vi "motor encoder.vi"(8 "Error In":errorcluster, 9 "motor select":T2, 10 "Reset":bool, 11 "FPGA VI Reference In":T1) -> (0 "error out":errorcluster, 1 "encoder":i32, 3 "FPGA VI Reference Out":T1)   [LabVIEW 2019, in "my FPGA lib.lvlib" / "motor.lvlib"]
uses:
  motor.lvlib
  motor enum.ctl
  FPGA/FPPGA.ctl
  <vilib>/Utility/error.llb/Error Cluster From Error Code.vi
  <vilib>/rvi/errors/niLvFpgaAdjustHostInterfaceError.vi
  <vilib>/rvi/interface/nirviReadWriteControl/nirviReadWriteControl.xnode
  NiFpgaLv.dll
  <vilib>/rvi/interface/Simulation/niFpgaSimulationCallBeginRW.vi
  my FPGA lib.lvlib
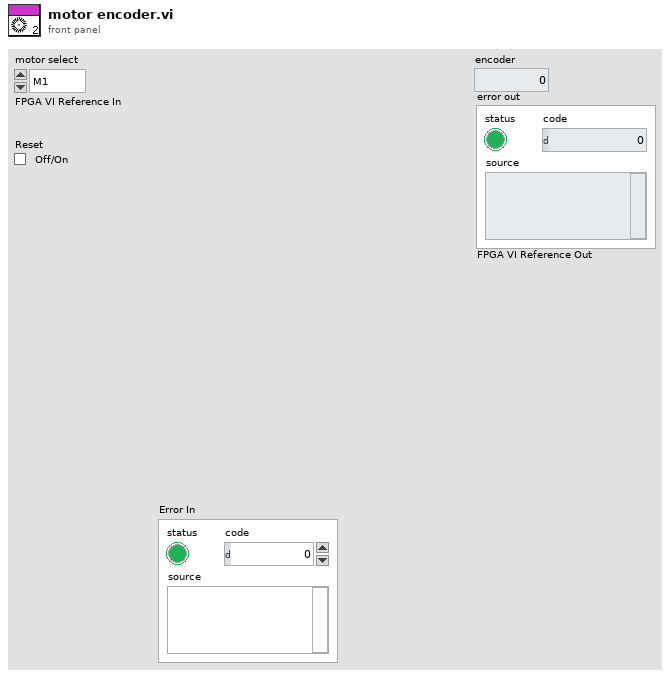
[diagram p1: front panel]
types:
  T1 = typedef "my FPGA lib.lvlib/FPPGA.ctl" = refnum<k20>
  T2 = typedef "my FPGA lib.lvlib/motor.lvlib/motor enum.ctl" = enum16{"M1", "M2", "M3", "M4"}
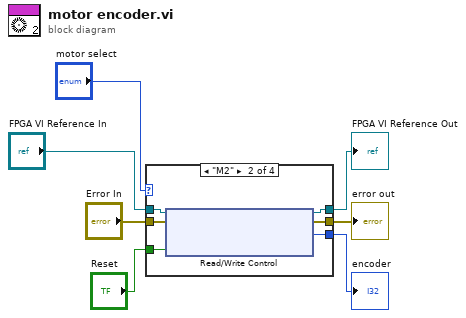
[diagram p0: block diagram]
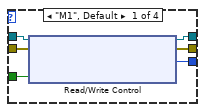
[diagram p2: hidden frame]
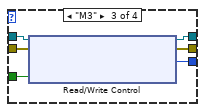
[diagram p3: hidden frame]
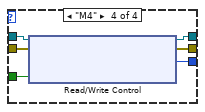
[diagram p4: hidden frame]
diagram:
  n1 = case shown="\"M2\"" "motor select" {
    tunnel: "FPGA VI Reference In" -> [w13 w19 w25 w31]
    tunnel: "Error In" -> [w12 w18 w24 w30]
    tunnel: "Reset" -> [w11 w17 w23 w29]
    tunnel: [w10 w16 w22 w28] -> w3
    tunnel: [w9 w15 w21 w27] -> w2
    tunnel: [w8 w14 w20 w26] -> w1
    frame "M1", Default {
      n2 = xnode "Read/Write Control"("FPGA VI Reference In"=w13, "error in"=w12, "Motor1.encoder_Reset"=w11) -> ("FPGA VI Reference Out"=w8:T1, "error out"=w9:errorcluster, "Motor1.encoder"=w10:i32)
    }
    frame "M2" {
      n3 = xnode "Read/Write Control"("FPGA VI Reference In"=w19, "error in"=w18, "Motor2.encoder_Reset"=w17) -> ("FPGA VI Reference Out"=w14:T1, "error out"=w15:errorcluster, "Motor2.encoder"=w16:i32)
    }
    frame "M3" {
      n4 = xnode "Read/Write Control"("FPGA VI Reference In"=w25, "error in"=w24, "Motor3.encoder_Reset"=w23) -> ("FPGA VI Reference Out"=w20:T1, "error out"=w21:errorcluster, "Motor3.encoder"=w22:i32)
    }
    frame "M4" {
      n5 = xnode "Read/Write Control"("FPGA VI Reference In"=w31, "error in"=w30, "Motor4.encoder_Reset"=w29) -> ("FPGA VI Reference Out"=w26:T1, "error out"=w27:errorcluster, "Motor4.encoder"=w28:i32)
    }
  }
  "encoder" <- w3
  "error out" <- w2
  "FPGA VI Reference Out" <- w1
